vi "SVPO Scale Voltage to EU (N Ch - N Info SGL WDT).vi"(7 "write waveform attributes? (T)":bool=TRUE, 10 "channel info":T1[](array[typedef]) {"pregain" format="%.2f"; "weighting filter" items=["Linear", "A-weighting", "B-weighting", "C-weighting", "ITU-R 468-4", "Dolby", "CCITT", "C-message", "Wb", "Wc", "Wd", "We", "Wf", "Wh", "Wj", "Wk", "Wm", "AES17 20 kHz lowpass", "AES17 40 kHz lowpass", "AES17 20 kHz highpass", "AES17 40 kHz highpass"]; "dB reference" format="%^.1e"; "engineering units" items=["custom..."=0, "V"=1, "A"=21, "C"=30, "pC"=31, "s"=32, "-"=29, "Pa"=2, "N"=20, "g"=3, "m/s^2"=4, "m/s"=5, "m"=6, "mm/s"=12, "mm"=13, "micron/s"=14, "micron"=15, "in/s^2"=7, "in/s"=8, "in"=9, "mil/s"=10, "mil"=11, "rad/s^2"=16, "rad/s"=17, "rad"=18, "deg/s^2"=26, "deg/s"=27, "deg"=28, "RPM"=22, "cycle/s^2"=23, "Hz"=24, "cycle"=25, "strain"=19]; "sensor sensitivity" format="%#_5f"}, 11 "signals [V]":waveform(sgl)[](array[waveform])) -> (3 "scaled signals [EU]":waveform(sgl)[](array[waveform]))   [LabVIEW 2017, in "SoundVib_Calibration.lvlib"]
doc: "Scales the single-precision <B>signal [V]</B> from volts to the engineering units (EU) you select. Scale signals to appropriate EU before applying limits, saving to disk, and performing measurement analyses. Use this VI on embedded targets that have limited computational resources. Wire data to the <B>signal [V]</B> input to determine the polymorphic instance to use or manually select the instance."
uses:
  <vilib>/addons/Sound and Vibration/svt_Calibration/SoundVib_Calibration.lvlib
  <vilib>/addons/_NISVFA/_Shared subVIs/Controls/svc_Channel Info.ctl
  <vilib>/addons/_NISVFA/_Shared subVIs/Controls/svc_Engineering Units Text Ring.ctl
  <vilib>/addons/_NISVFA/_Shared subVIs/Controls/svc_Weighting Filter Text Ring.ctl
  <vilib>/addons/_NISVFA/_Shared subVIs/Common/svc_Set SV Channel Info (SGL).vi
  <vilib>/addons/_NISVFA/_Shared subVIs/Common/svc_Set SV Channel Info (variant).vi
  <vilib>/addons/_NISVFA/_Shared subVIs/Common/SVL Set dB Reference (variant).vi
  <vilib>/addons/_NISVFA/_Shared subVIs/Common/svc_Engineering Units to Unit Label.vi
  <vilib>/addons/_NISVFA/_Shared subVIs/Common/svc_Set dB ref if Pascal.vi
  <vilib>/addons/_NISVFA/_Shared subVIs/Common/svc_Compute Scale Factor to Convert V to EU.vi
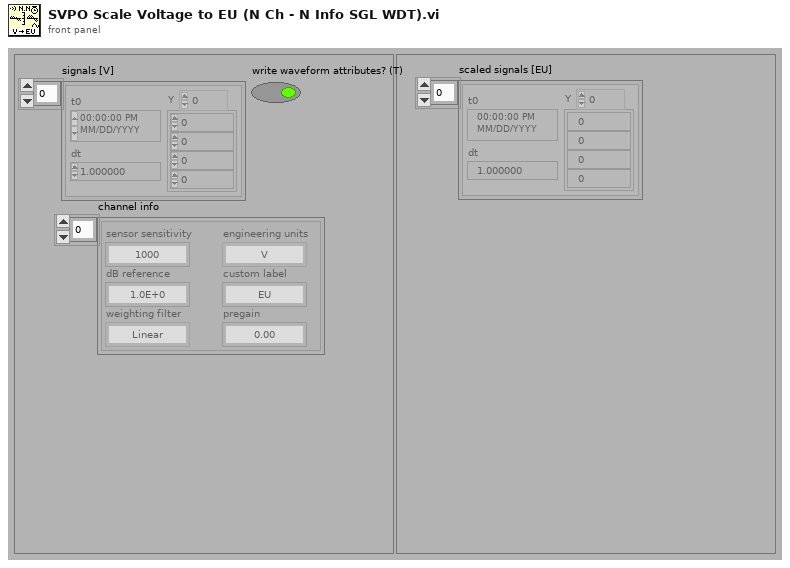
[diagram p1: front panel]
types:
  T1 = typedef "svc_Channel Info.ctl" = cluster{"sensor sensitivity":dbl, "engineering units":T2, "dB reference":dbl, "custom label":string, "weighting filter":T3, "pregain":dbl}
  T2 = typedef "svc_Engineering Units Text Ring.ctl" = u16
  T3 = typedef "svc_Weighting Filter Text Ring.ctl" = u16
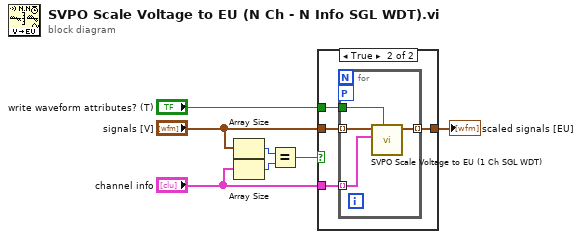
[diagram p0: block diagram]
diagram:
  n1 = Array Size(array="signals [V]") -> (size(s)=w5:i32)
  n2 = Array Size(array="channel info") -> (size(s)=w4:i32)
  n3 = Equal?(x=w5, y=w4) -> (x = y?=w1:bool)
  n4 = case shown="True" w1 {
    tunnel: "write waveform attributes? (T)" -> [_ w11]
    tunnel: [_ w10] -> w6
    tunnel: "signals [V]" -> [_ w9]
    tunnel: "channel info" -> [_ w8]
    frame False {
    }
    frame True {
      n5 = for {
        tunnel: w9 -> [w15] mode=indexing
        tunnel: w8 -> [w14] mode=indexing
        tunnel: [w13] -> w10 mode=indexing
        tunnel: w11 -> [w12]
        workers-P: _ -> [_]
        n6 = call <vilib>:"SVPO Scale Voltage to EU (1 Ch SGL WDT).vi"("write waveform attributes? (T)"=w12, "channel info"=w14, "signal [V]"=w15) -> ("scaled signal [EU]"=w13:waveform(sgl))  [unwired: 8 in]
      }
    }
  }
  "scaled signals [EU]" <- w6
